vi "Test-ProvePilot.vi"(8 "error in":errorcluster, 10 "Boiler Configuration":T3) -> (3 "MHL Data":T1)   [LabVIEW 2017, in "Controller.lvlib"]
uses:
  Controller.lvlib
  controls/MHL UI Data.ctl
  controls/MHL Status.ctl
  Boiler/Boiler.lvlib
  support/Message Queue/Message Queue.lvlib
panel:
  in  "Flame Threshold":u32
  out "error out":errorcluster
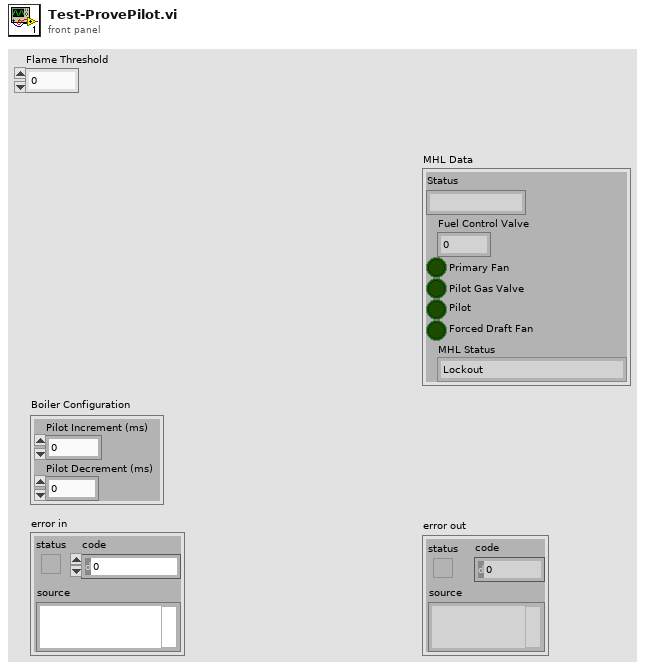
[diagram p1: front panel]
types:
  T1 = typedef "MHL UI Data.ctl" = cluster{"Status":string, "Fuel Control Valve":u32, "Primary Fan":bool, "Pilot Gas Valve":bool, "Pilot":bool, "Forced Draft Fan":bool, "MHL Status":T2}
  T2 = typedef "MHL Status.ctl" = enum16{"Lockout", "Ready", "Pre-Purge", "Pre-Purge Complete", "Pilot On", "Boiler Running", "Shutdown", "Purge"}
  T3 = cluster{"Pilot Increment (ms)":u32, "Pilot Decrement (ms)":u32}
  T4 = enum16{"open", "replace", "create", "open or create", "replace or create", "replace or create with confirmation"}
  T5 = typedef "Message Queue.lvlib/All Message Queues.ctl" = cluster{"MHL":refnum<queue>, "Boiler Controller":refnum<queue>, "Boiler":refnum<queue>}
  T6 = typedef "Notifiers.ctl" = cluster{"Handshake":refnum<notifier>, "Flame Level":refnum<notifier>, "Controller Exit":refnum<notifier>, "Boiler Exit":refnum<notifier>}
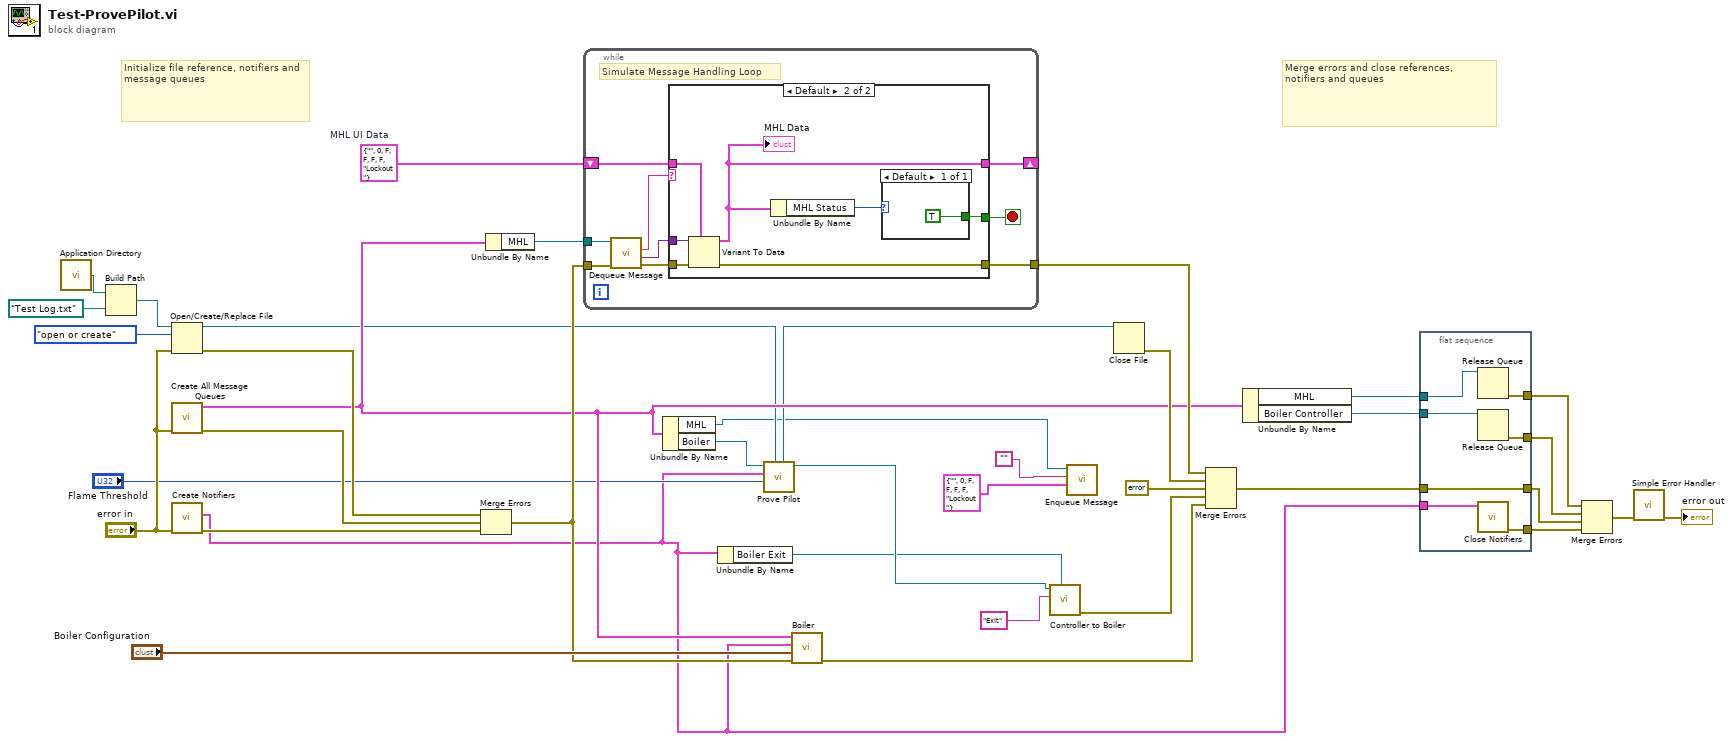
[diagram p0: block diagram]
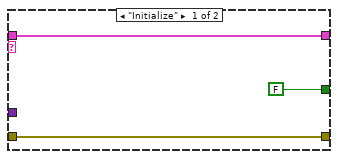
[diagram p2: hidden frame]
diagram:
  w27 = T1 {"Status"="", "Fuel Control Valve"=0, "Primary Fan"=FALSE, "Pilot Gas Valve"=FALSE, "Pilot"=FALSE, "Forced Draft Fan"=FALSE, "MHL Status"=enum."Lockout"}  # MHL UI Data
  # "Merge errors and close references, notifiers and queues"
  # "Initialize file reference, notifiers and message queues"
  n1 = call <vilib>:"Application Directory.vi"() -> ("Application Directory"=w36:path)
  n2 = Build Path(base path=w36, name or relative path=path "Test Log.txt") -> (appended path=w34:path)
  n3 = Open/Create/Replace File(file path (use dialog)=w34, error in="error in", operation (0:open)=T4."open or create") -> (refnum out=w8:refnum<file>, error out=w32:errorcluster)  [unwired: 3 in, 1 out]
  n4 = call "Create All Message Queues.vi"("error in (no error)"="error in") -> ("error out"=w37:errorcluster, "Message Queues out"=w12:T5)  [unwired: 9 in]
  n5 = call "Create Notifiers.vi"("error constant"="error in") -> ("error out"=w38:errorcluster, "output cluster"=w2:T6)  [unwired: 9 in]
  n6 = Merge Errors(w32, w37, w38) -> (w28:errorcluster)
  n7 = Unbundle By Name(w12) -> ("MHL"=w29:refnum<queue>)
  n8 = while {
    tunnel: w29 -> [w47]
    tunnel: w28 -> [w46]
    shift-right: [w43] -> _
    shift-left: w27 -> [w44]
    tunnel: [w40] -> w23
    stop <- w39 stop-if-true
    # "Simulate Message Handling Loop"
    n9 = call "Dequeue Message.vi"("error in (no error)"=w46, "Message Queue"=w47) -> ("error out"=w41:errorcluster, "Message Data"=w45:variant, "Message"=w42:string)  [unwired: 6 in, 1 out]
    n10 = case shown="Default" w42 {
      tunnel: w41 -> [w48 w57]
      tunnel: w45 -> [_ w56]
      tunnel: w44 -> [w50 w55]
      tunnel: [w50 w54] -> w43
      tunnel: [FALSE w52] -> w39
      tunnel: [w48 w51] -> w40
      frame "Initialize" {
      }
      frame Default {
        n11 = Variant To Data(error in=w57, type=w55, Variant=w56) -> (data=w54:T1, error out=w51:errorcluster)
        "MHL Data" <- w54
        n12 = Unbundle By Name(w54) -> ("MHL Status"=w53:T2)
        n13 = case shown="Default" w53 {
          tunnel: [TRUE] -> w52
          frame Default {
          }
        }
      }
    }
  }
  n14 = Unbundle By Name(w12) -> ("MHL"=w6:refnum<queue>, "Boiler"=w10:refnum<queue>)
  n15 = Unbundle By Name(w2) -> ("Boiler Exit"=w1:refnum<notifier>)
  n16 = call "Prove Pilot.vi"("Log File Refnum in"=w8, "Flame Threshold"="Flame Threshold", "Notifiers in"=w2, "Boiler Queue in"=w10) -> ("Boiler Queue out"=w3:refnum<queue>, "Log File Refnum out"=w7:refnum<file>)  [unwired: 4 in, 2 out]
  n17 = call "Boiler.vi"("error in"=w28, "Boiler Configuration"="Boiler Configuration", "Notifiers"=w2, "Message Queues"=w12) -> ("error out"=w14:errorcluster)  [unwired: 7 in]
  n18 = call "Controller to Boiler.vi"("Notifier"=w1, "Message"="Exit", "Boiler Queue in"=w3) -> ("error out"=w13:errorcluster)  [unwired: 6 in, 2 out]
  n19 = call "Enqueue Message.vi"("Message Data"=T1 {"Status"="", "Fuel Control Valve"=0, "Primary Fan"=FALSE, "Pilot Gas Valve"=FALSE, "Pilot"=FALSE, "Forced Draft Fan"=FALSE, "MHL Status"=enum."Lockout"} ("MHL UI Data"), "Message"="", "Message Queue"=w6) -> ()  [unwired: 7 in, 2 out]
  n20 = Close File(refnum=w7) -> (error out=w24:errorcluster)  [unwired: 1 in, 1 out]
  n21 = Merge Errors(w23, w24, errorcluster {"status"=FALSE, "code"=0, "source"=""} ("error in"), w13, w14) -> (w15:errorcluster)
  n22 = Unbundle By Name(w12) -> ("MHL"=w25:refnum<queue>, "Boiler Controller"=w26:refnum<queue>)
  n23 = flat-sequence {
    tunnel: w26 -> [w65]
    tunnel: w25 -> [w64]
    tunnel: [w63] -> w21
    tunnel: [w62] -> w20
    tunnel: [w61] -> w17
    tunnel: [w60] -> w16
    tunnel: w15 -> [w60]
    tunnel: w2 -> [w59]
    frame #0 {
      n24 = Release Queue(queue=w64) -> (error out=w62:errorcluster)  [unwired: 2 in, 2 out]
      n25 = Release Queue(queue=w65) -> (error out=w63:errorcluster)  [unwired: 2 in, 2 out]
      n26 = call "Close Notifiers.vi"("output cluster"=w59) -> ("error out"=w61:errorcluster)  [unwired: 10 in]
    }
  }
  n27 = Merge Errors(w20, w21, w16, w17) -> (w19:errorcluster)
  n28 = call <vilib>:"Simple Error Handler.vi"("error in (no error)"=w19) -> ("error out"=→"error out":errorcluster)  [unwired: 4 in, 4 out]
